vi "Calc EEG Volts.vi"(10 "Gain":u8=24, 11 "Array":u8[](array[numeric]) format="%x") -> (3 "Volts":dbl)   [LabVIEW 2019, in "Acquisition.lvlib"]
uses:
  Acquisition.lvlib
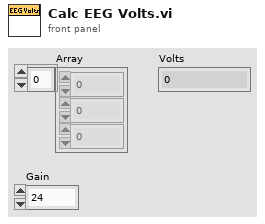
[diagram p1: front panel]
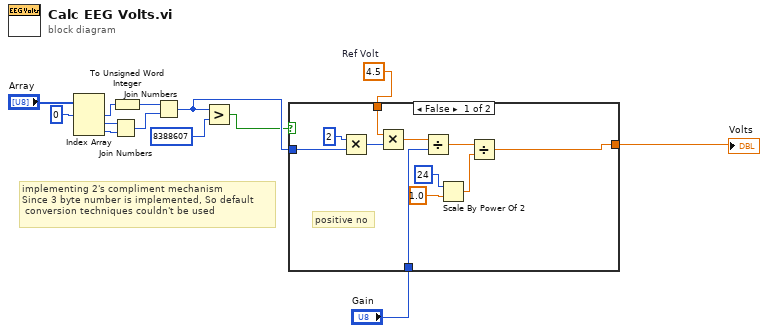
[diagram p0: block diagram]
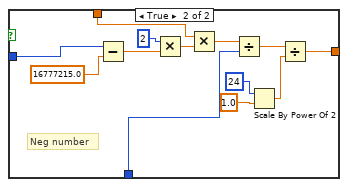
[diagram p2: hidden frame]
diagram:
  w11 = sgl 4.5  # Ref Volt
  # "implementing 2's compliment mechanism\nSince 3 byte number is implemented, So default\n conversion techniques couldn't be used"
  n1 = Index Array(array="Array", index #1=0 ("index")) -> (element #1=w1:u8, element #2=w3:u8, element #3=w4:u8)  [unwired: 2 in]
  n2 = Join Numbers(hi=w3, lo=w4) -> ((hi.lo)=w2:u16)
  n3 = To Unsigned Word Integer(number=w1) -> (unsigned 16bit integer=w7:u16)
  n4 = Join Numbers(hi=w7, lo=w2) -> ((hi.lo)=w10:u32)
  n5 = Greater?(x=w10, y=u32 8388607) -> (0:w9:bool)
  n6 = case shown="False" w9 {
    tunnel: w10 -> [w17 w36]
    tunnel: [w16 w25] -> w13
    tunnel: w11 -> [w15 w27]
    tunnel: "Gain" -> [w14 w26]
    frame False {
      # "positive no"
      n7 = Multiply(x=u32 2, y=w17) -> (x*y=w19:u32)
      n8 = Multiply(x=w15, y=w19) -> (x*y=w20:sgl)
      n9 = Divide(x=w20, y=w14) -> (x/y=w21:sgl)
      n10 = Scale By Power Of 2(n=i16 24, x=1.0) -> (x*2^n=w24:dbl)
      n11 = Divide(x=w21, y=w24) -> (x/y=w16:dbl)
    }
    frame True {
      # "Neg number"
      n12 = Subtract(x=w36, y=16777215.0) -> (x-y=w28:dbl)
      n13 = Multiply(x=u32 2, y=w28) -> (x*y=w30:dbl)
      n14 = Multiply(x=w27, y=w30) -> (x*y=w31:dbl)
      n15 = Divide(x=w31, y=w26) -> (x/y=w32:dbl)
      n16 = Scale By Power Of 2(n=i16 24, x=1.0) -> (x*2^n=w35:dbl)
      n17 = Divide(x=w32, y=w35) -> (x/y=w25:dbl)
    }
  }
  "Volts" <- w13
